vi "ziSubscribe.vi"(3 "error in":errorcluster, 4 "Path ()":string, 5 "Handle In":T1 {"Handle" format="0x%08x"; "Conn" format="0x%08x"}) -> (0 "error out":errorcluster, 2 "Handle Out":T1 {"Handle" format="0x%08x"; "Conn" format="0x%08x"})   [LabVIEW 2009, in "Zurich Instruments LabOne.lvlib"]
doc: "Subscribes to nodes so that whenever the value of the node changes the new value can be polled using ziPollDataEx.vi. By using wildcards or by using a <b>Path</b> that is not a leaf node but contains sub nodes, more than one node can be subscribed to with one function call."
uses:
  <instrlib>/Zurich Instruments LabOne/Zurich Instruments LabOne.lvlib
  <instrlib>/Zurich Instruments LabOne/Public/ziTypeHandle.ctl
  <instrlib>/Zurich Instruments LabOne/Private/ziLV64.dll
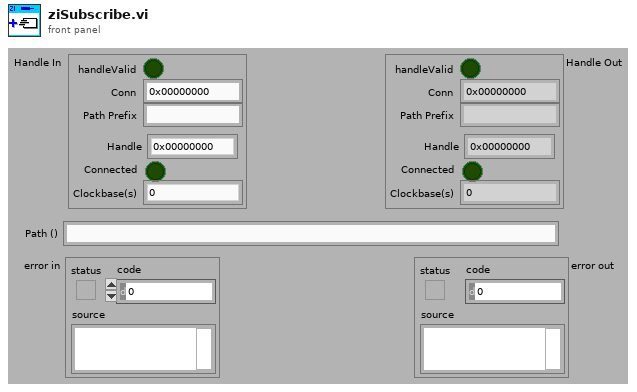
[diagram p1: front panel]
types:
  T1 = typedef "Zurich Instruments LabOne.lvlib/ziTypeHandle.ctl" = cluster{"handleValid":bool, "Conn":u64, "Path Prefix":string, "Handle":u64, "Connected":bool, "Clockbase(s)":dbl}
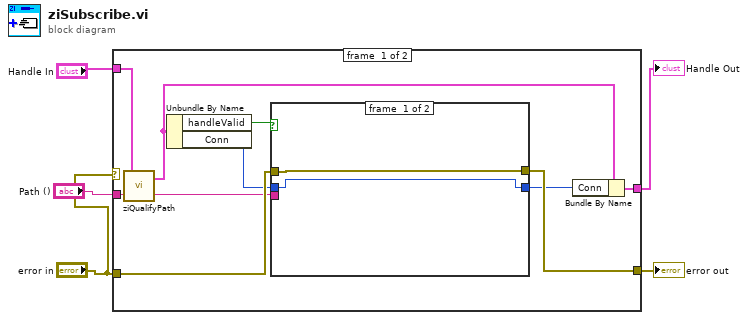
[diagram p0: block diagram]
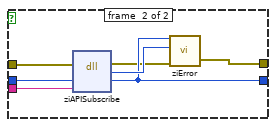
[diagram p2: hidden frame]
diagram:
  n1 = case shown="No Error" "error in" {
    tunnel: "error in" -> [w15 w25]
    tunnel: [w14 w25] -> w5
    tunnel: [w11 w26] -> w4
    tunnel: "Path ()" -> [w10 _]
    tunnel: "Handle In" -> [w8 w26]
    frame #0 {
      n2 = call <instrlib>:"ziQualifyPath.vi"("Path In"=w10, "Handle In"=w8) -> ("Path Out"=w9:string, "Handle Out"=w7:T1)
      n3 = Unbundle By Name(w7) -> ("handleValid"=w13:bool, "Conn"=w12:u64)
      n4 = case shown="True" w13 {
        tunnel: w15 -> [w17 w24]
        tunnel: w12 -> [w16 w23]
        tunnel: [w16 w20] -> w6
        tunnel: [w17 w18] -> w14
        tunnel: w9 -> [_ w22]
        frame #0 {
        }
        frame #1 {
          n5 = dll-call lib="C:/Program Files/National Instruments/LabVIEW 2009/instr.lib/Zurich Instruments LabOne/Private/ziLV*.*" fn="ziAPISubscribe"(error in=w24, "Conn"=w23, "Path"=w22) -> (error out=w19:errorcluster, "return type"=w21:u32, "Conn"=w20:u64)  [unwired: 3 in, 1 out]
          n6 = call <instrlib>:"ziError.vi"("Conn"=w20, "ziErrorCode"=w21, "Error In"=w19) -> ("Error Out"=w18:errorcluster)  [unwired: 2 in, 1 out]
        }
      }
      n7 = Bundle By Name(cluster=w7, "Conn"=w6) -> (w11:T1)
    }
    frame #1 {
    }
  }
  "error out" <- w5
  "Handle Out" <- w4
